vi "cylindrical_sample_setup.vi"(10 "D (mm)":dbl=10.0, 11 "H (mm)":dbl=2.0) -> (1 "Result":dbl, 3 "spreadsheet string":string)   [LabVIEW 2011]
uses:
  <vilib>/express/express arith-compare/Formula/XNode/ExpressFormulaBlockNode.xnode
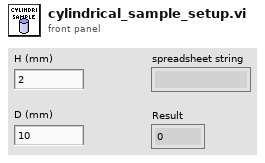
[diagram p1: front panel]
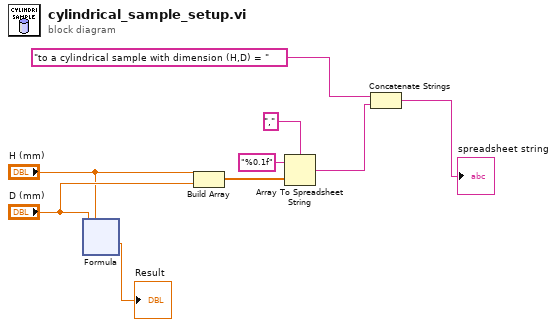
[diagram p0: block diagram]
diagram:
  n1 = xnode "Formula"("D"="D (mm)", "H"="H (mm)") -> ("Result"=→"Result":dbl)  [unwired: 1 in, 1 out]
  n2 = Build Array("H (mm)", "D (mm)") -> (w6:dbl[])
  n3 = Array To Spreadsheet String(delimiter (Tab)=",", array=w6, 3:"%0.1f" ("format string")) -> (spreadsheet string=w2:string)
  n4 = Concatenate Strings("to a cylindrical sample with dimension (H,D) = " ("string"), w2) -> (→"spreadsheet string":string)
